vi "XBox Manipulator.vi"() -> (0 "Secondary Controller":T1)   [LabVIEW 2014]
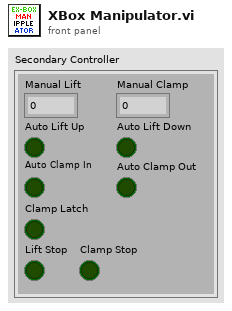
[diagram p1: front panel]
types:
  T1 = cluster{"Manual Lift":dbl, "Manual Clamp":dbl, "Auto Lift Up":bool, "Auto Lift Down":bool, "Auto Clamp In":bool, "Auto Clamp Out":bool, "Clamp Latch":bool, "Lift Stop":bool, "Clamp Stop":bool}
  T2 = cluster{"Buttons":cluster{"A":bool, "B":bool, "X":bool, "Y":bool, "L Bumper":bool, "R Bumper":bool, "Back":bool, "Start":bool, "LStick":bool, "RStick":bool}, "Axes":cluster{"Left Stick":cluster{"X":dbl, "Y":dbl}, "Right Stick":cluster{"X":dbl, "Y":dbl}, "L Trigger":dbl, "R Trigger":dbl}}
  T3 = cluster{dbl, "X":dbl, "Y":bool, "A":bool, "X":bool, "B":bool, "R Bumper":bool, bool, bool}
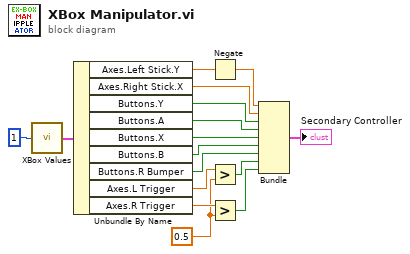
[diagram p0: block diagram]
diagram:
  w3 = 0.5 ("y")
  n1 = call "XBox Values.vi"("Index"=1) -> ("XBox"=w15:T2)
  n2 = Unbundle By Name(w15) -> ("Axes.Left Stick.Y"=w8:dbl, "Axes.Right Stick.X"=w6:dbl, "Buttons.Y"=w14:bool, "Buttons.A"=w13:bool, "Buttons.X"=w12:bool, "Buttons.B"=w11:bool, "Buttons.R Bumper"=w9:bool, "Axes.L Trigger"=w5:dbl, "Axes.R Trigger"=w4:dbl)
  n3 = Negate(x=w8) -> (-x=w7:dbl)
  n4 = Greater?(x=w5, y=w3) -> (0:w2:bool)
  n5 = Greater?(x=w4, y=w3) -> (0:w1:bool)
  n6 = Bundle(w7, "X"=w6, "Y"=w14, "A"=w13, "X"=w12, "B"=w11, "R Bumper"=w9, w2, w1) -> (→"Secondary Controller":T3)  [unwired: 1 in]
